vi "Get BLISS_Get List of Servers (SubVI).vi"(8 "error in (no error)":errorcluster, 9 "Intial Server List":string[](array[string]), 10 "Initial Action":T1=enum."Open File") -> (0 "error out":errorcluster, 1 "Server List":string[](array[string]), 3 "Message Out":string)   [LabVIEW 2020]
uses:
  Get BLISS_Enum Control.ctl
  Get BLISS_Global Error Codes.vi
  MC5e Gobal_Variables.vi
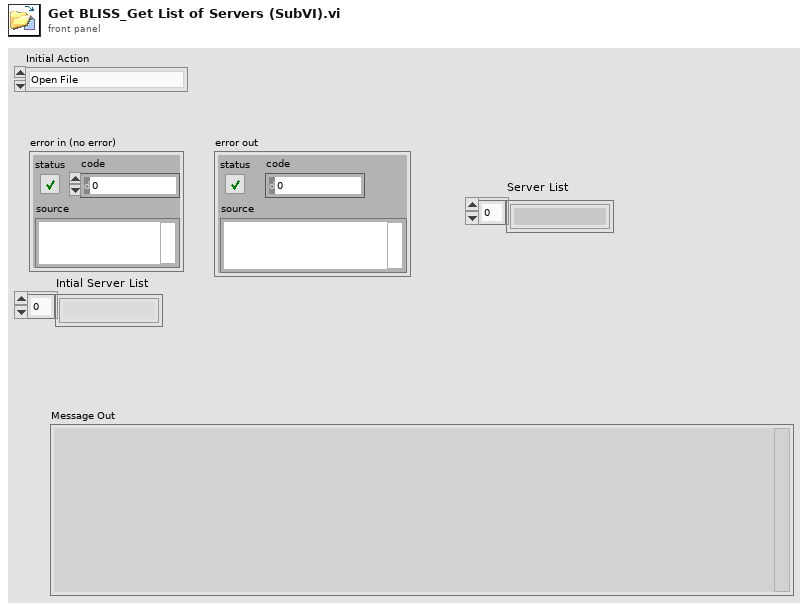
[diagram p1: front panel]
types:
  T1 = typedef "Get BLISS_Enum Control.ctl" = enum16{"Exit", "Open File", "Ask for File", "Use Default List", "Give Examples", "Create Array"}
  T2 = enum16{"open", "replace", "create", "open or create", "replace or create", "replace or create with confirmation"}
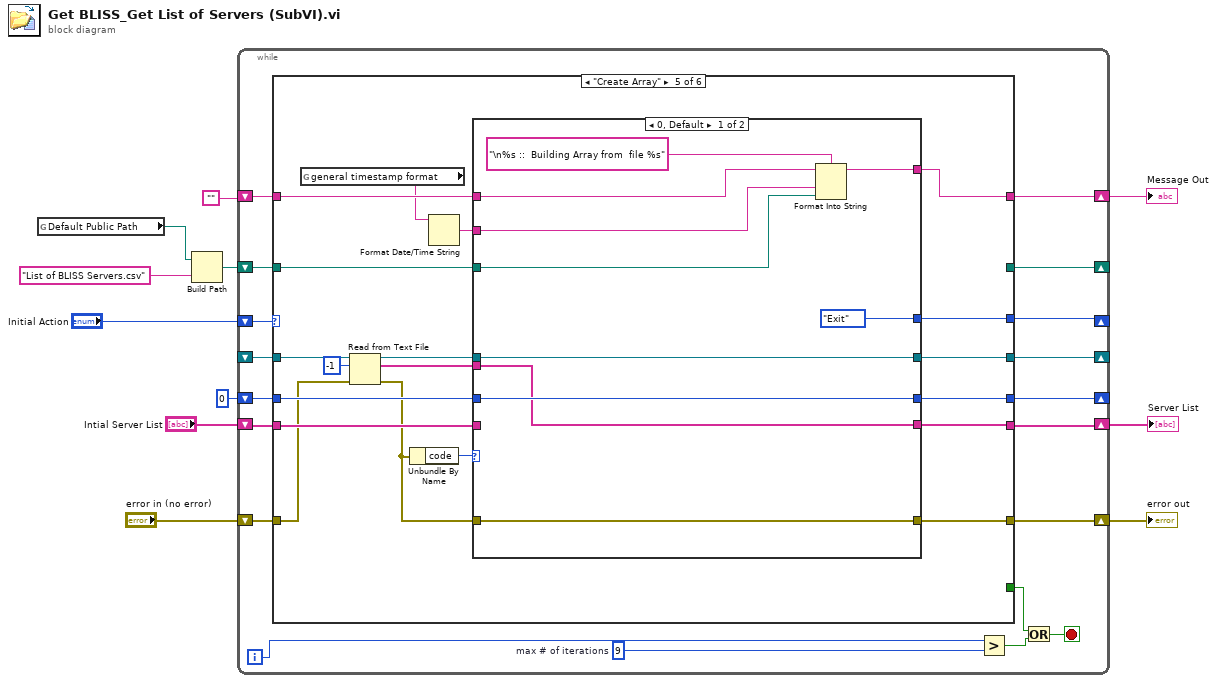
[diagram p0: block diagram]
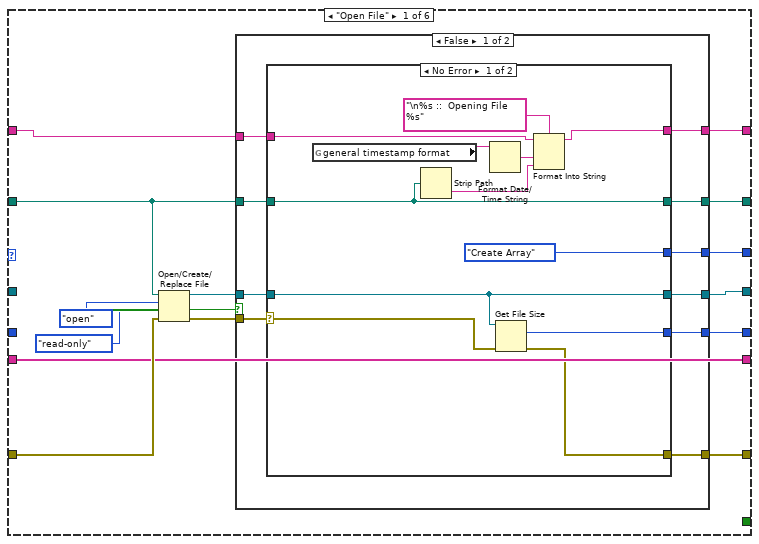
[diagram p2: hidden frame]
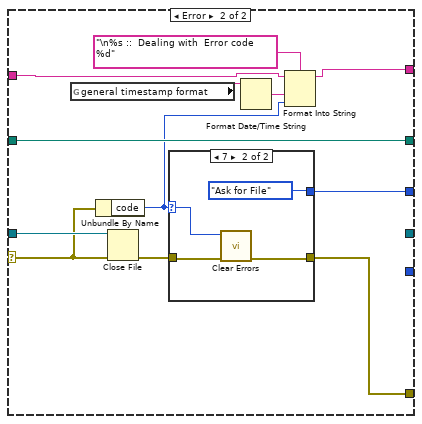
[diagram p3: hidden frame]
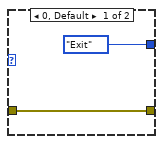
[diagram p4: hidden frame]
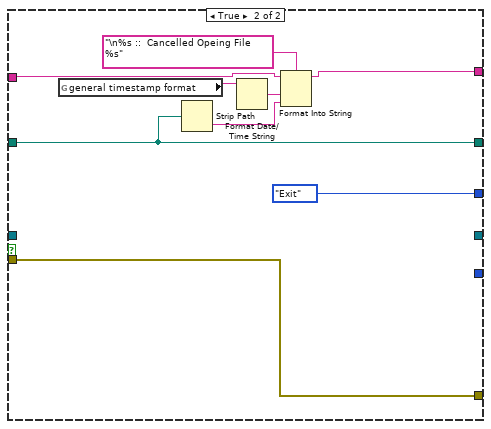
[diagram p5: hidden frame]
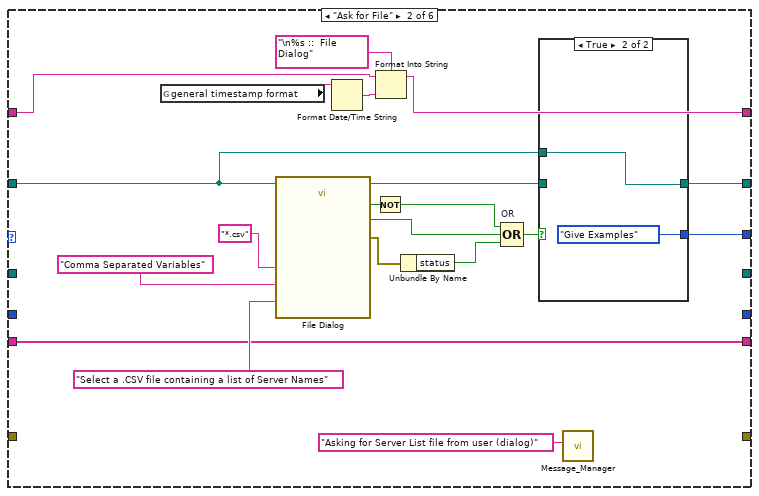
[diagram p6: hidden frame]
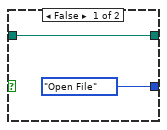
[diagram p7: hidden frame]
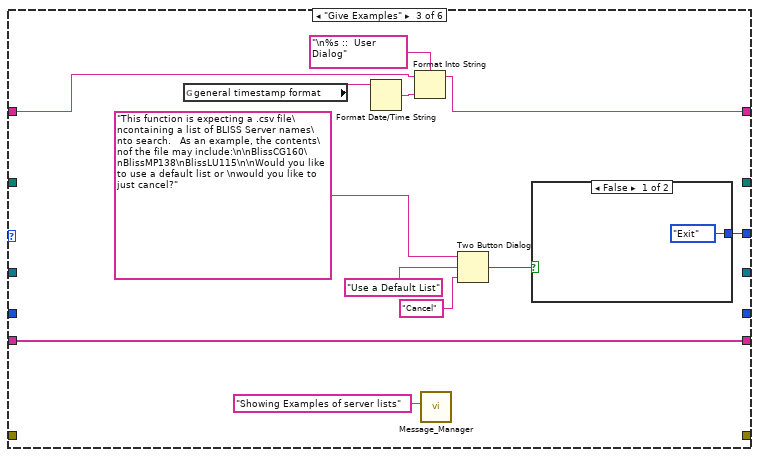
[diagram p8: hidden frame]
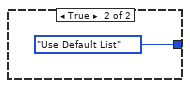
[diagram p9: hidden frame]
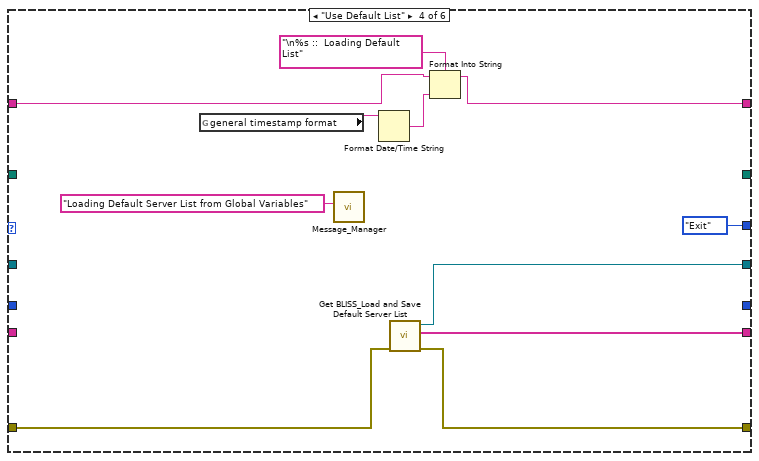
[diagram p10: hidden frame]
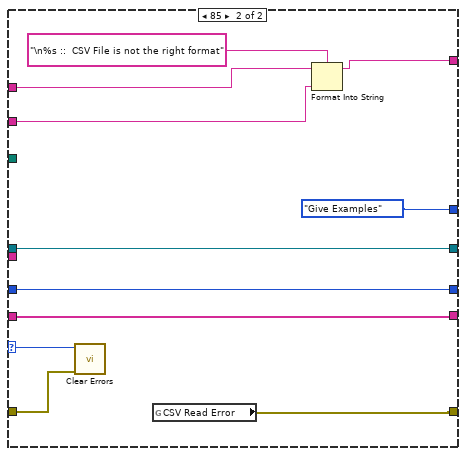
[diagram p11: hidden frame]
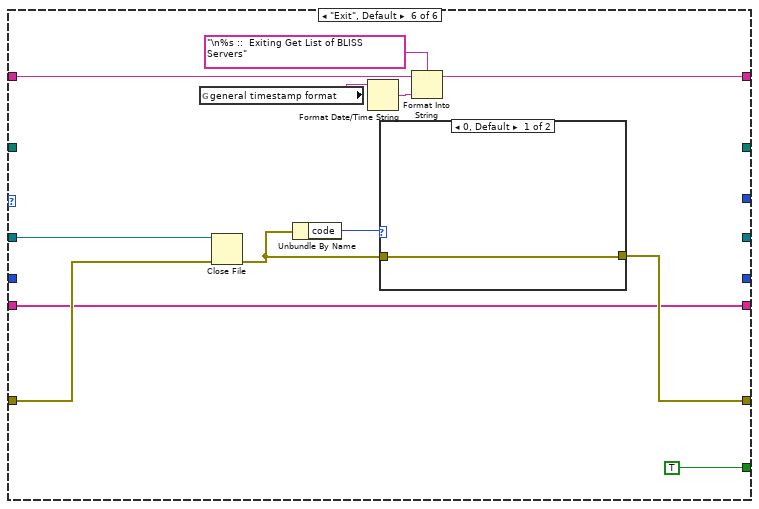
[diagram p12: hidden frame]
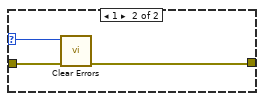
[diagram p13: hidden frame]
diagram:
  n1 = global read "MC5e Gobal_Variables.vi" "Default Public Path"() -> (w1:path)
  n2 = Build Path(base path=w1, name or relative path="List of BLISS Servers.csv") -> (appended path=w9:path)
  n3 = while {
    shift-right: [w21] -> _
    shift-left: "Initial Action" -> [w30]
    shift-right: [w20] -> _
    shift-left: w9 -> [w24]
    shift-right: [w23] -> w8
    shift-left: "error in (no error)" -> [w22]
    shift-right: [w19] -> _
    shift-left: _ -> [w18]
    shift-right: [w17] -> w6
    shift-left: "" -> [w16]
    shift-right: [w15] -> _
    shift-left: i64 0 ("size (in bytes)") -> [w14]
    shift-right: [w12] -> w2
    shift-left: "Intial Server List" -> [w13]
    i -> [w29]
    stop <- w26 stop-if-true
    w28 = 9  # max # of iterations
    n4 = case shown="\"Create Array\"" w30 {
      tunnel: [_ _ _ _ _ TRUE] -> w25
      tunnel: w24 -> [w36 w102 _ _ w146 _]
      tunnel: [w40 _ _ w136 w160 w186] -> w23
      tunnel: w22 -> [w39 _ _ w138 w151 w189]
      tunnel: [w38 w103 w126 Get_BLISS_Enum_Control."Exit" w157 _] -> w21
      tunnel: [w37 w105 _ _ _ _] -> w20
      tunnel: [w35 _ _ w137 w161 _] -> w19
      tunnel: w18 -> [_ _ _ _ w152 w190]
      tunnel: [w33 w98 w122 w140 w156 w191] -> w17
      tunnel: w16 -> [w34 w99 w123 w141 w159 w193]
      tunnel: [w32 _ _ _ w153 _] -> w15
      tunnel: w14 -> [_ _ _ _ w154 _]
      tunnel: w13 -> [w31 w97 w121 _ w158 w185]
      tunnel: [w31 w97 w121 w135 w145 w185] -> w12
      frame "Open File" {
        n5 = Open/Create/Replace File(file path (use dialog)=w36, error in=w39, operation (0:open)=T2."open", access (0:read/write)=enum16{"read/write", "read-only", "write-only"}."read-only") -> (refnum out=w44:refnum<file>, cancelled=w45:bool, error out=w43:errorcluster)  [unwired: 2 in]
        n6 = case shown="False" w45 {
          tunnel: w44 -> [w53 _]
          tunnel: w43 -> [w55 w94]
          tunnel: [w54 _] -> w35
          tunnel: [w52 w94] -> w40
          tunnel: [w51 Get_BLISS_Enum_Control."Exit"] -> w38
          tunnel: [w50 w88] -> w37
          tunnel: w36 -> [w49 w88]
          tunnel: w34 -> [w48 w90]
          tunnel: [w47 w89] -> w33
          tunnel: [w46 _] -> w32
          frame False {
            n7 = case shown="No Error" w55 {
              selector: w55 -> [w61 w78]
              tunnel: [w62 _] -> w54
              tunnel: w53 -> [w62 w79]
              tunnel: [w60 w75] -> w52
              tunnel: [Get_BLISS_Enum_Control."Create Array" w77] -> w51
              tunnel: [w58 w76] -> w50
              tunnel: w49 -> [w58 w76]
              tunnel: w48 -> [w64 w70]
              tunnel: [w63 w69] -> w47
              tunnel: [w59 _] -> w46
              frame No Error {
                n8 = global read "MC5e Gobal_Variables.vi" "general timestamp format"() -> (w56:string)
                n9 = Strip Path(path=w58) -> (name=w57:string)  [unwired: 1 out]
                n10 = Format Date/Time String(time format string (%c)=w56) -> (date/time string=w65:string)  [unwired: 2 in]
                n11 = Get File Size(file=w62, error in=w61) -> (size (in bytes)=w59:i64, 0:w60:errorcluster)  [unwired: 1 out]
                n12 = Format Into String(format string="\n%s ::  Opening File %s", initial string=w64, w65, w57) -> (resulting string=w63:string)  [unwired: 1 in, 1 out]
              }
              frame Error {
                n13 = global read "MC5e Gobal_Variables.vi" "general timestamp format"() -> (w68:string)
                n14 = Unbundle By Name(w78) -> ("code"=w71:i32)
                n15 = Close File(refnum=w79, error in=w78) -> (error out=w74:errorcluster)  [unwired: 1 out]
                n16 = case shown="7" w71 {
                  selector: w71 -> [_ w82]
                  tunnel: [Get_BLISS_Enum_Control."Exit" Get_BLISS_Enum_Control."Ask for File"] -> w77
                  tunnel: [w80 w83] -> w75
                  tunnel: w74 -> [w80 w84]
                  frame 0, Default {
                  }
                  frame 7 {
                    n17 = call <vilib>:"Clear Errors.vi"("error in (no error)"=w84, "specific error code to clear (0: all)"=w82) -> ("error out"=w83:errorcluster)  [unwired: 4 in, 1 out]
                  }
                }
                n18 = Format Date/Time String(time format string (%c)=w68) -> (date/time string=w72:string)  [unwired: 2 in]
                n19 = Format Into String(format string="\n%s ::  Dealing with  Error code %d", initial string=w70, w72, w71) -> (resulting string=w69:string)  [unwired: 1 in, 1 out]
              }
            }
          }
          frame True {
            n20 = global read "MC5e Gobal_Variables.vi" "general timestamp format"() -> (w86:string)
            n21 = Strip Path(path=w88) -> (name=w87:string)  [unwired: 1 out]
            n22 = Format Date/Time String(time format string (%c)=w86) -> (date/time string=w91:string)  [unwired: 2 in]
            n23 = Format Into String(format string="\n%s ::  Cancelled Opeing File %s", initial string=w90, w91, w87) -> (resulting string=w89:string)  [unwired: 1 in, 1 out]
          }
        }
      }
      frame "Ask for File" {
        n24 = global read "MC5e Gobal_Variables.vi" "general timestamp format"() -> (w96:string)
        n25 = call "File Dialog"("start path"=w102, "prompt"="Select a .CSV file containing a list of Server Names" ("name or relative path"), "pattern (all files)"="*.csv" ("name or relative path"), "pattern label"="Comma Separated Variables" ("name or relative path")) -> ("selected path"=w104:path, "exists"=w110:bool, "cancelled"=w108:bool, "error out"=w111:errorcluster)  [unwired: 8 in]
        n26 = Format Date/Time String(time format string (%c)=w96) -> (date/time string=w100:string)  [unwired: 2 in]
        n27 = Not(x=w110) -> (.not. x?=w109:bool)
        n28 = Format Into String(format string="\n%s ::  File Dialog", initial string=w99, w100) -> (resulting string=w98:string)  [unwired: 1 in, 1 out]
        n29 = Unbundle By Name(w111) -> ("status"=w107:bool)
        n30 = Compound Arithmetic op=OR "OR"(w109, w108, w107) -> (w106:bool)
        n31 = case shown="True" w106 {
          tunnel: [w116 w117] -> w105
          tunnel: w104 -> [w116 _]
          tunnel: [Get_BLISS_Enum_Control."Open File" Get_BLISS_Enum_Control."Give Examples"] -> w103
          tunnel: w102 -> [_ w117]
          frame False {
          }
          frame True {
          }
        }
        n32 = call "Message_Manager.vi"("New Entry"="Asking for Server List file from user (dialog)") -> ()  [unwired: 5 in, 6 out]
      }
      frame "Give Examples" {
        n33 = global read "MC5e Gobal_Variables.vi" "general timestamp format"() -> (w120:string)
        n34 = Format Date/Time String(time format string (%c)=w120) -> (date/time string=w124:string)  [unwired: 2 in]
        n35 = Format Into String(format string="\n%s ::  User Dialog", initial string=w123, w124) -> (resulting string=w122:string)  [unwired: 1 in, 1 out]
        n36 = call "Message_Manager.vi"("New Entry"="Showing Examples of server lists") -> ()  [unwired: 5 in, 6 out]
        n37 = Two Button Dialog(message="This function is expecting a .csv file\ncontaining a list of BLISS Server names\nto search.   As an example, the contents\nof the file may include:\n\nBlissCG160\nBlissMP138\nBlissLU115\n\nWould you like to use a default list or \nwould you like to just cancel?", 1:"Cancel" ("T button name (\"OK\")"), 2:"Use a Default List" ("F button name (\"Cancel\")")) -> (T button?=w127:bool)
        n38 = case shown="False" w127 {
          tunnel: [Get_BLISS_Enum_Control."Exit" Get_BLISS_Enum_Control."Use Default List"] -> w126
          frame False {
          }
          frame True {
          }
        }
      }
      frame "Use Default List" {
        n39 = global read "MC5e Gobal_Variables.vi" "general timestamp format"() -> (w134:string)
        n40 = call "Message_Manager.vi"("New Entry"="Loading Default Server List from Global Variables") -> ()  [unwired: 5 in, 6 out]
        n41 = Format Date/Time String(time format string (%c)=w134) -> (date/time string=w143:string)  [unwired: 2 in]
        n42 = call "Get BLISS_Load and Save Default Server List.vi"("error in (no error)"=w138) -> ("error out"=w136:errorcluster, "Server Names (Dup)"=w135:string[], "File Ref Out"=w137:refnum<file>)  [unwired: 8 in]
        n43 = Format Into String(format string="\n%s ::  Loading Default List", initial string=w141, w143) -> (resulting string=w140:string)  [unwired: 1 in, 1 out]
      }
      frame "Create Array" {
        n44 = global read "MC5e Gobal_Variables.vi" "general timestamp format"() -> (w144:string)
        n45 = Read from Text File(file (use dialog)=w152, count=-1, error in=w151) -> (refnum out=w148:refnum<file>, text=w147:string[], error out=w150:errorcluster)  [unwired: 1 in, 1 out]
        n46 = Unbundle By Name(w150) -> ("code"=w162:i32)
        n47 = Format Date/Time String(time format string (%c)=w144) -> (date/time string=w155:string)  [unwired: 2 in]
        n48 = case shown="0, Default" w162 {
          selector: w162 -> [_ w183]
          tunnel: [w172 w174] -> w160
          tunnel: w150 -> [w172 w182]
          tunnel: w148 -> [w171 w181]
          tunnel: [w171 w181] -> w161
          tunnel: w159 -> [w168 w177]
          tunnel: w158 -> [_ w173]
          tunnel: w147 -> [w163 _]
          tunnel: [w163 w173] -> w145
          tunnel: [Get_BLISS_Enum_Control."Exit" Get_BLISS_Enum_Control."Give Examples"] -> w157
          tunnel: w154 -> [w165 w175]
          tunnel: [w167 w176] -> w156
          tunnel: w155 -> [w166 w178]
          tunnel: [w165 w175] -> w153
          tunnel: w146 -> [w164 _]
          frame 0, Default {
            n49 = Format Into String(format string="\n%s ::  Building Array from  file %s", initial string=w168, w166, w164) -> (resulting string=w167:string)  [unwired: 1 in, 1 out]
          }
          frame 85 {
            n50 = call <vilib>:"Clear Errors.vi"("error in (no error)"=w182, "specific error code to clear (0: all)"=w183) -> ()  [unwired: 4 in, 2 out]
            n51 = global read "Get BLISS_Global Error Codes.vi" "CSV Read Error"() -> (w174:errorcluster)
            n52 = Format Into String(format string="\n%s ::  CSV File is not the right format", initial string=w177, w178) -> (resulting string=w176:string)  [unwired: 1 in, 1 out]
          }
        }
      }
      frame "Exit", Default {
        n53 = global read "MC5e Gobal_Variables.vi" "general timestamp format"() -> (w184:string)
        n54 = Close File(refnum=w190, error in=w189) -> (error out=w187:errorcluster)  [unwired: 1 out]
        n55 = Unbundle By Name(w187) -> ("code"=w188:i32)
        n56 = Format Date/Time String(time format string (%c)=w184) -> (date/time string=w192:string)  [unwired: 2 in]
        n57 = case shown="0, Default" w188 {
          selector: w188 -> [_ w198]
          tunnel: [w196 w199] -> w186
          tunnel: w187 -> [w196 w197]
          frame 0, Default {
          }
          frame 1 {
            n58 = call <vilib>:"Clear Errors.vi"("error in (no error)"=w197, "specific error code to clear (0: all)"=w198) -> ("error out"=w199:errorcluster)  [unwired: 4 in, 1 out]
          }
        }
        n59 = Format Into String(format string="\n%s ::  Exiting Get List of BLISS Servers", initial string=w193, w192) -> (resulting string=w191:string)  [unwired: 1 in, 1 out]
      }
    }
    n60 = Greater?(x=w29, y=w28) -> (0:w27:bool)
    n61 = Or(x=w25, y=w27) -> (x .or. y?=w26:bool)
  }
  "error out" <- w8
  "Message Out" <- w6
  "Server List" <- w2
